vi "DAQmx Read (Digital 1D Wfm NChan 1Samp).vi"(0 "task/channels in":refnum<k21>, 9 "timeout":dbl=10.0 format="%0.2f", 11 "error in":errorcluster) -> (4 "task out":refnum<k21>, 6 "data":digitalwaveform[](array[waveform]), 15 "error out":errorcluster)   [LabVIEW 2020]
doc: "Reads a waveform that contains a single sample from each channel in a task that contains one or more digital input channels."
uses:
  nilvaiu.dll
panel:
  # "channel"
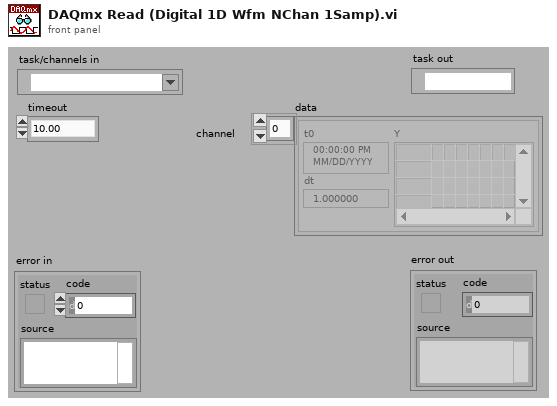
[diagram p1: front panel]
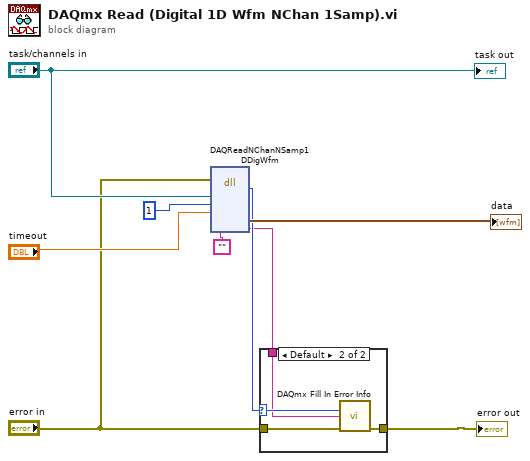
[diagram p0: block diagram]
diagram:
  n1 = dll-call lib="nilvaiu.*" fn="DAQReadNChanNSamp1DDigWfm"(error in="error in", "taskID"="task/channels in", "samplesPerChannel"=1, "timeout"="timeout", "extendedErrorInfo"="") -> (w5:i32, "data"=→"data":digitalwaveform[], "extendedErrorInfo"=w3:string)  [unwired: 4 in, 4 out]
  n2 = case shown="Default" w5 {
    selector: w5 -> [_ w12]
    tunnel: "error in" -> [w10 w14]
    tunnel: [w10 w13] -> w9
    tunnel: w3 -> [_ w11]
    frame 0 {
    }
    frame Default {
      n3 = call "DAQmx Fill In Error Info.vi"("status code"=w12, "extended error info"=w11, "error in"=w14) -> ("error out"=w13:errorcluster)  [unwired: 1 in, 11 out]
    }
  }
  "error out" <- w9
  "task out" <- "task/channels in"
